vi "QUEUE.vi"() -> ()   [LabVIEW 2013]
panel:
  out "Waveform Chart":dbl(graph)
  in  "stop":bool
  in  "send":bool
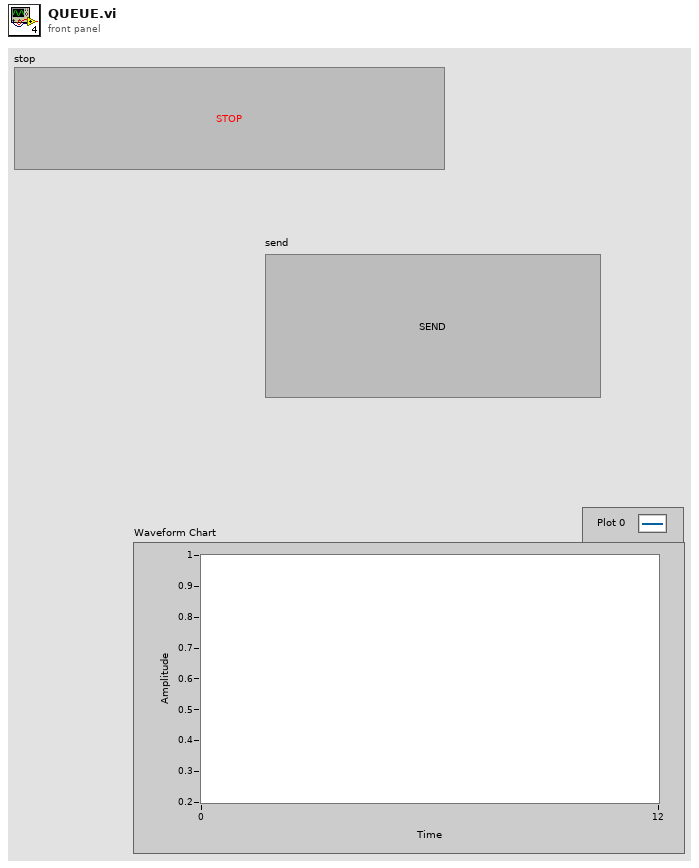
[diagram p1: front panel]
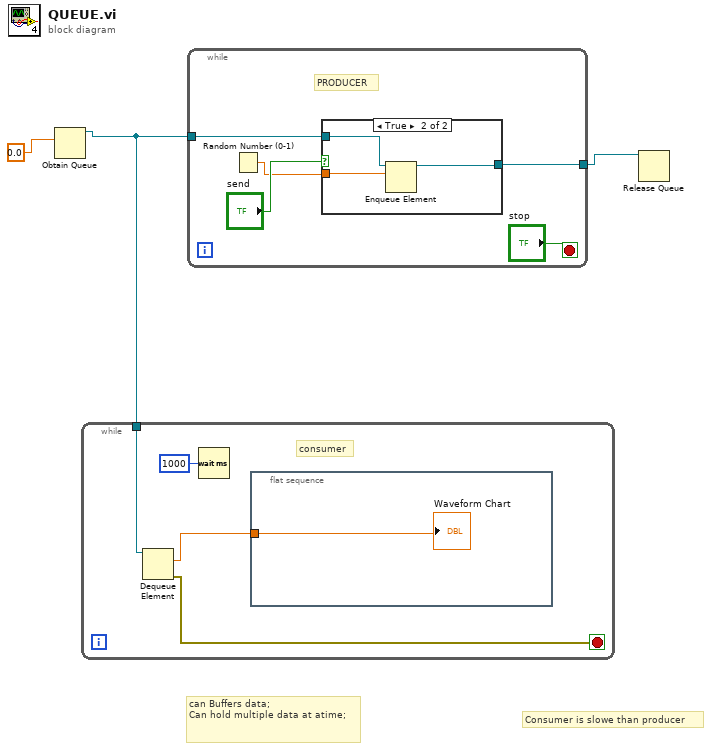
[diagram p0: block diagram]
diagram:
  # "Consumer is slowe than producer"
  # "can Buffers data;\nCan hold multiple data at atime;"
  n1 = Obtain Queue(element data type=0.0) -> (queue out=w3:refnum<queue>)  [unwired: 4 in, 2 out]
  n2 = while {
    tunnel: w3 -> [w7]
    stop <- w6 stop-if-true
    # "consumer"
    n3 = Dequeue Element(queue=w7) -> (element=w5:dbl, error out=w6:errorcluster)  [unwired: 2 in, 2 out]
    n4 = Wait (ms)(milliseconds to wait=u32 1000) -> ()  [unwired: 1 out]
    n5 = flat-sequence {
      tunnel: w5 -> [w8]
      frame #0 {
        "Waveform Chart" <- w8
      }
    }
  }
  n6 = while {
    tunnel: w3 -> [w11]
    tunnel: [w10] -> w1
    stop <- "stop" stop-if-true
    # "PRODUCER"
    n7 = Random Number (0-1)() -> (number: 0 to 1=w9:dbl)
    n8 = case shown="True" "send" {
      tunnel: w11 -> [w14 w17]
      tunnel: [w14 w16] -> w10
      tunnel: w9 -> [_ w15]
      frame False {
      }
      frame True {
        n9 = Enqueue Element(queue=w17, element=w15) -> (queue out=w16:refnum<queue>)  [unwired: 2 in, 2 out]
      }
    }
  }
  n10 = Release Queue(queue=w1) -> ()  [unwired: 2 in, 3 out]
